vi "Double FFT Mesurament (Max Bin detection - Control - Windowing - Graph) test.vi"() -> ()   [LabVIEW 2014]
uses:
  <vilib>/Platform/TimedLoop/XDataNode/timing_clust.ctl
  <vilib>/Platform/TimedLoop/XDataNode/nitl_modes.ctl
  <vilib>/Platform/TimedLoop/XDataNode/wakeup.ctl
  <vilib>/rvi/Analysis/measure/FFT/simModelSupport/niFPGA FFT Streaming Sim Properties.ctl
  <vilib>/rvi/Analysis/measure/FFT/simModelSupport/niFPGA FFT Sim Stream Group Properties.ctl
  <vilib>/rvi/Analysis/measure/FFT/simModelSupport/niFPGA FFT Sim Types.ctl
  <vilib>/rvi/Analysis/measure/FFT/simModelSupport/niFpgaFFTSimArithmeticProperties.ctl
  <vilib>/rvi/Analysis/measure/FFT/simModelSupport/niFpgaFFTSimDfxp.ctl
  <vilib>/fxp/LVFixedPointQuantizationPolicyTypeDef.ctl
  <vilib>/rvi/Analysis/measure/FFT/XNode/niFpgaFFTButterflyDelays.ctl
  <vilib>/rvi/Emulation/niFpgaSctlEmulationGetInTimedLoop.vi
  <vilib>/rvi/Emulation/niFpgaEmulationReportErrorSimple.vi
  <vilib>/rvi/Emulation/niFpgaGetClockAttributes.vi
  <vilib>/rvi/Emulation/niFpgaCriticalErrorInLSC.vi
  <vilib>/rvi/Emulation/niFpgaEmulationIsFPGAContextNoSignature.vi
  <vilib>/rvi/errors/niFpgaSetErrorForExecOnDevCompSimple.vi
  <vilib>/rvi/eio/common/nirviEmuReportErrorAndStop.vi
  <vilib>/rvi/DataTransferAndStorage/Container/Common/niFpgaContainerGetUniqueNameForEmu.vi
  <vilib>/rvi/FIFO/Fifo_Resource/nirvififoEmulationSetSize.vi
  <vilib>/rvi/FIFO/Fifo_Resource/nirviFifoEmulationQueueMgr.vi
  <instcachedir>/0/nirviFifoEmulationQueueMgr_E5CAEC123FF24DC58D834DCA3CDAA9B5.lvgen/nirviFifoEmulationQueueMgr_E5CAEC123FF24DC58D834DCA3CDAA9B5_005.vi
  <vilib>/Utility/error.llb/Clear Errors.vi
  <vilib>/rvi/FIFO/Fifo_Resource/nirvififoEmulationCreateLock.vi
  <vilib>/rvi/Emulation/niFpgaProcessEmulError.vi
  <vilib>/rvi/FIFO/Fifo_Resource/nirvififoEmulationObtainLock.vi
  <vilib>/rvi/FIFO/Fifo_Resource/nirvififoEmulationReleaseLock.vi
  <vilib>/rvi/occurrence/nirviWaitOnOccurrenceBase.vi
  <vilib>/rvi/errors/nirviReportUnexpectedCaseInternalError.vi
  <vilib>/rvi/errors/nirviReportUnexpectedCaseInternalError (U32).vi
  <instcachedir>/0/nirviFifoEmulationQueueMgr_E5CAEC123FF24DC58D834DCA3CDAA9B5.lvgen/nirviFifoEmulationQueueMgr_E5CAEC123FF24DC58D834DCA3CDAA9B5_004.vi
  <vilib>/rvi/interface/RandomDataEmulation/niFpgaRandomDataHandleErrors.vi
  <vilib>/rvi/Memory/Memory_Emulation/niFpgaMemoryEmulationCacheClearOnFirstRun.vi
  <vilib>/rvi/Memory/Memory_Emulation/nirvimemoryEmulationManagerCache_MakeExclusive.vi
  <vilib>/rvi/Memory/Memory_Emulation/niFpgaMemoryEmulationValidateCache.vi
  <vilib>/rvi/Memory/Memory_Emulation/nirvimemoryEmulationManagerCache_InsertValue.vi
  <vilib>/rvi/Memory/Memory_Emulation/nirvimemoryEmulationManagerCache_ReleaseExclusive.vi
  <vilib>/rvi/Memory/Memory_Emulation/nirvimemoryEmulationManagerCache_GetValue.vi
  <vilib>/rvi/Memory/Memory_Emulation/nirvimemoryEmulationManagerCache_SetValue.vi
  <vilib>/rvi/FIFO/Fifo_Resource/nirvififoEmulationDetermineInputValidOut.vi
  <vilib>/rvi/Memory/Memory_Emulation/nirvimemoryFastEmulation.vi
  <vilib>/rvi/Memory/Memory_Emulation/nirvimemoryEmulation.vi
  <vilib>/rvi/Analysis/measure/FFT/simModelSupport/niFpgaFFTSimModelStreamingCore.vi
  <vilib>/rvi/eio/common/nirviEmuTemplateMethod_errors.vi
  <vilib>/Platform/TimedLoop/XDataNode/XDataNode.xnode
  <vilib>/rvi/DataTransferAndStorage/Container/XNode/niFpgaContainer.xnode
  <vilib>/rvi/FIFO/Fifo_Resource/nirvififoEmulationRead.vi
  <vilib>/rvi/interface/RandomDataEmulation/nirviRandomDataFpgaReadWriteTemplate.vi
  <vilib>/rvi/DataTransferAndStorage/Register/Emulation/niFpgaRegisterEmulation.vi
  <vilib>/rvi/FIFO/Fifo_Resource/nirvififoEmulationWrite.vi
  <vilib>/rvi/FIFO/Fifo_Resource/nirvififoEmulationGetNumberOfElementsToWrite.vi
  <vilib>/rvi/Analysis/measure/FFT/XNode/niFpgaFFT.xnode
  <vilib>/eio/EIOMethodNode/EIOMethodNode.xnode
  <vilib>/Platform/TimedLoop/XDataNode/XDNodeRunTimeDep.lvlib
panel:
  in  "snapshot":bool
  in  "first bin":i32=4
  in  "last bin":i32=251
  in  "lower limit 2":u32=682
  in  "lower limit 1":u32=57
  in  "upper limit 2":u32=1194
  in  "upper limit 1":u32=569
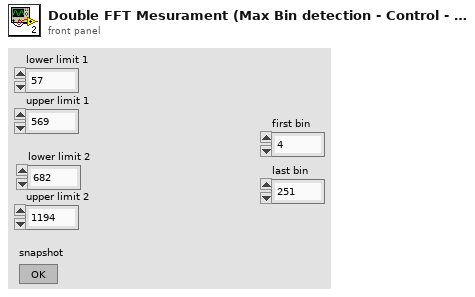
[diagram p1: front panel]
types:
  T1 = typedef "XDNodeRunTimeDep.lvlib/timing_clust.ctl" = cluster{"Expected End [f-1]":u64, "Actual End [f-1]":u64, "Finished Late? [f-1]":bool, "Expected End [i-1]":u64, "Actual End [i-1]":u64, "Finished Late? [i-1]":bool, "Expected Start [i]":u64, "Actual Start [i]":u64, "Expected Start [f]":u64, "Actual Start [f]":u64, "Source Name":string, "Structure Name":string, "Period":i64, "Deadline":i64, "Offset":i64, "Start":i64, "Priority":i32, "Timeout":i32, "Mode":T2, "Wakeup Reason":T3, "Error":errorcluster, "Source Type":string, "Secondary Source Type":string, "Global End Time":u64, "Global Start Time":u64, "Frame Duration":u64, "Iteration Duration":u64, "Assigned CPU":i32, "I/O Scan Engine Mode":u32}
  T2 = typedef "XDNodeRunTimeDep.lvlib/nitl_modes.ctl" = enum32{"No Change", "Process missed periods, maintain original phase", "Discard missed periods, maintain original phase", "Process missed periods, ignore original phase", "Discard missed periods, ignore original phase"}
  T3 = typedef "XDNodeRunTimeDep.lvlib/wakeup.ctl" = enum32{"Normal", "Aborted", "Asynchronous wakeup", "Timing source error", "Timed loop error", "Timeout"}
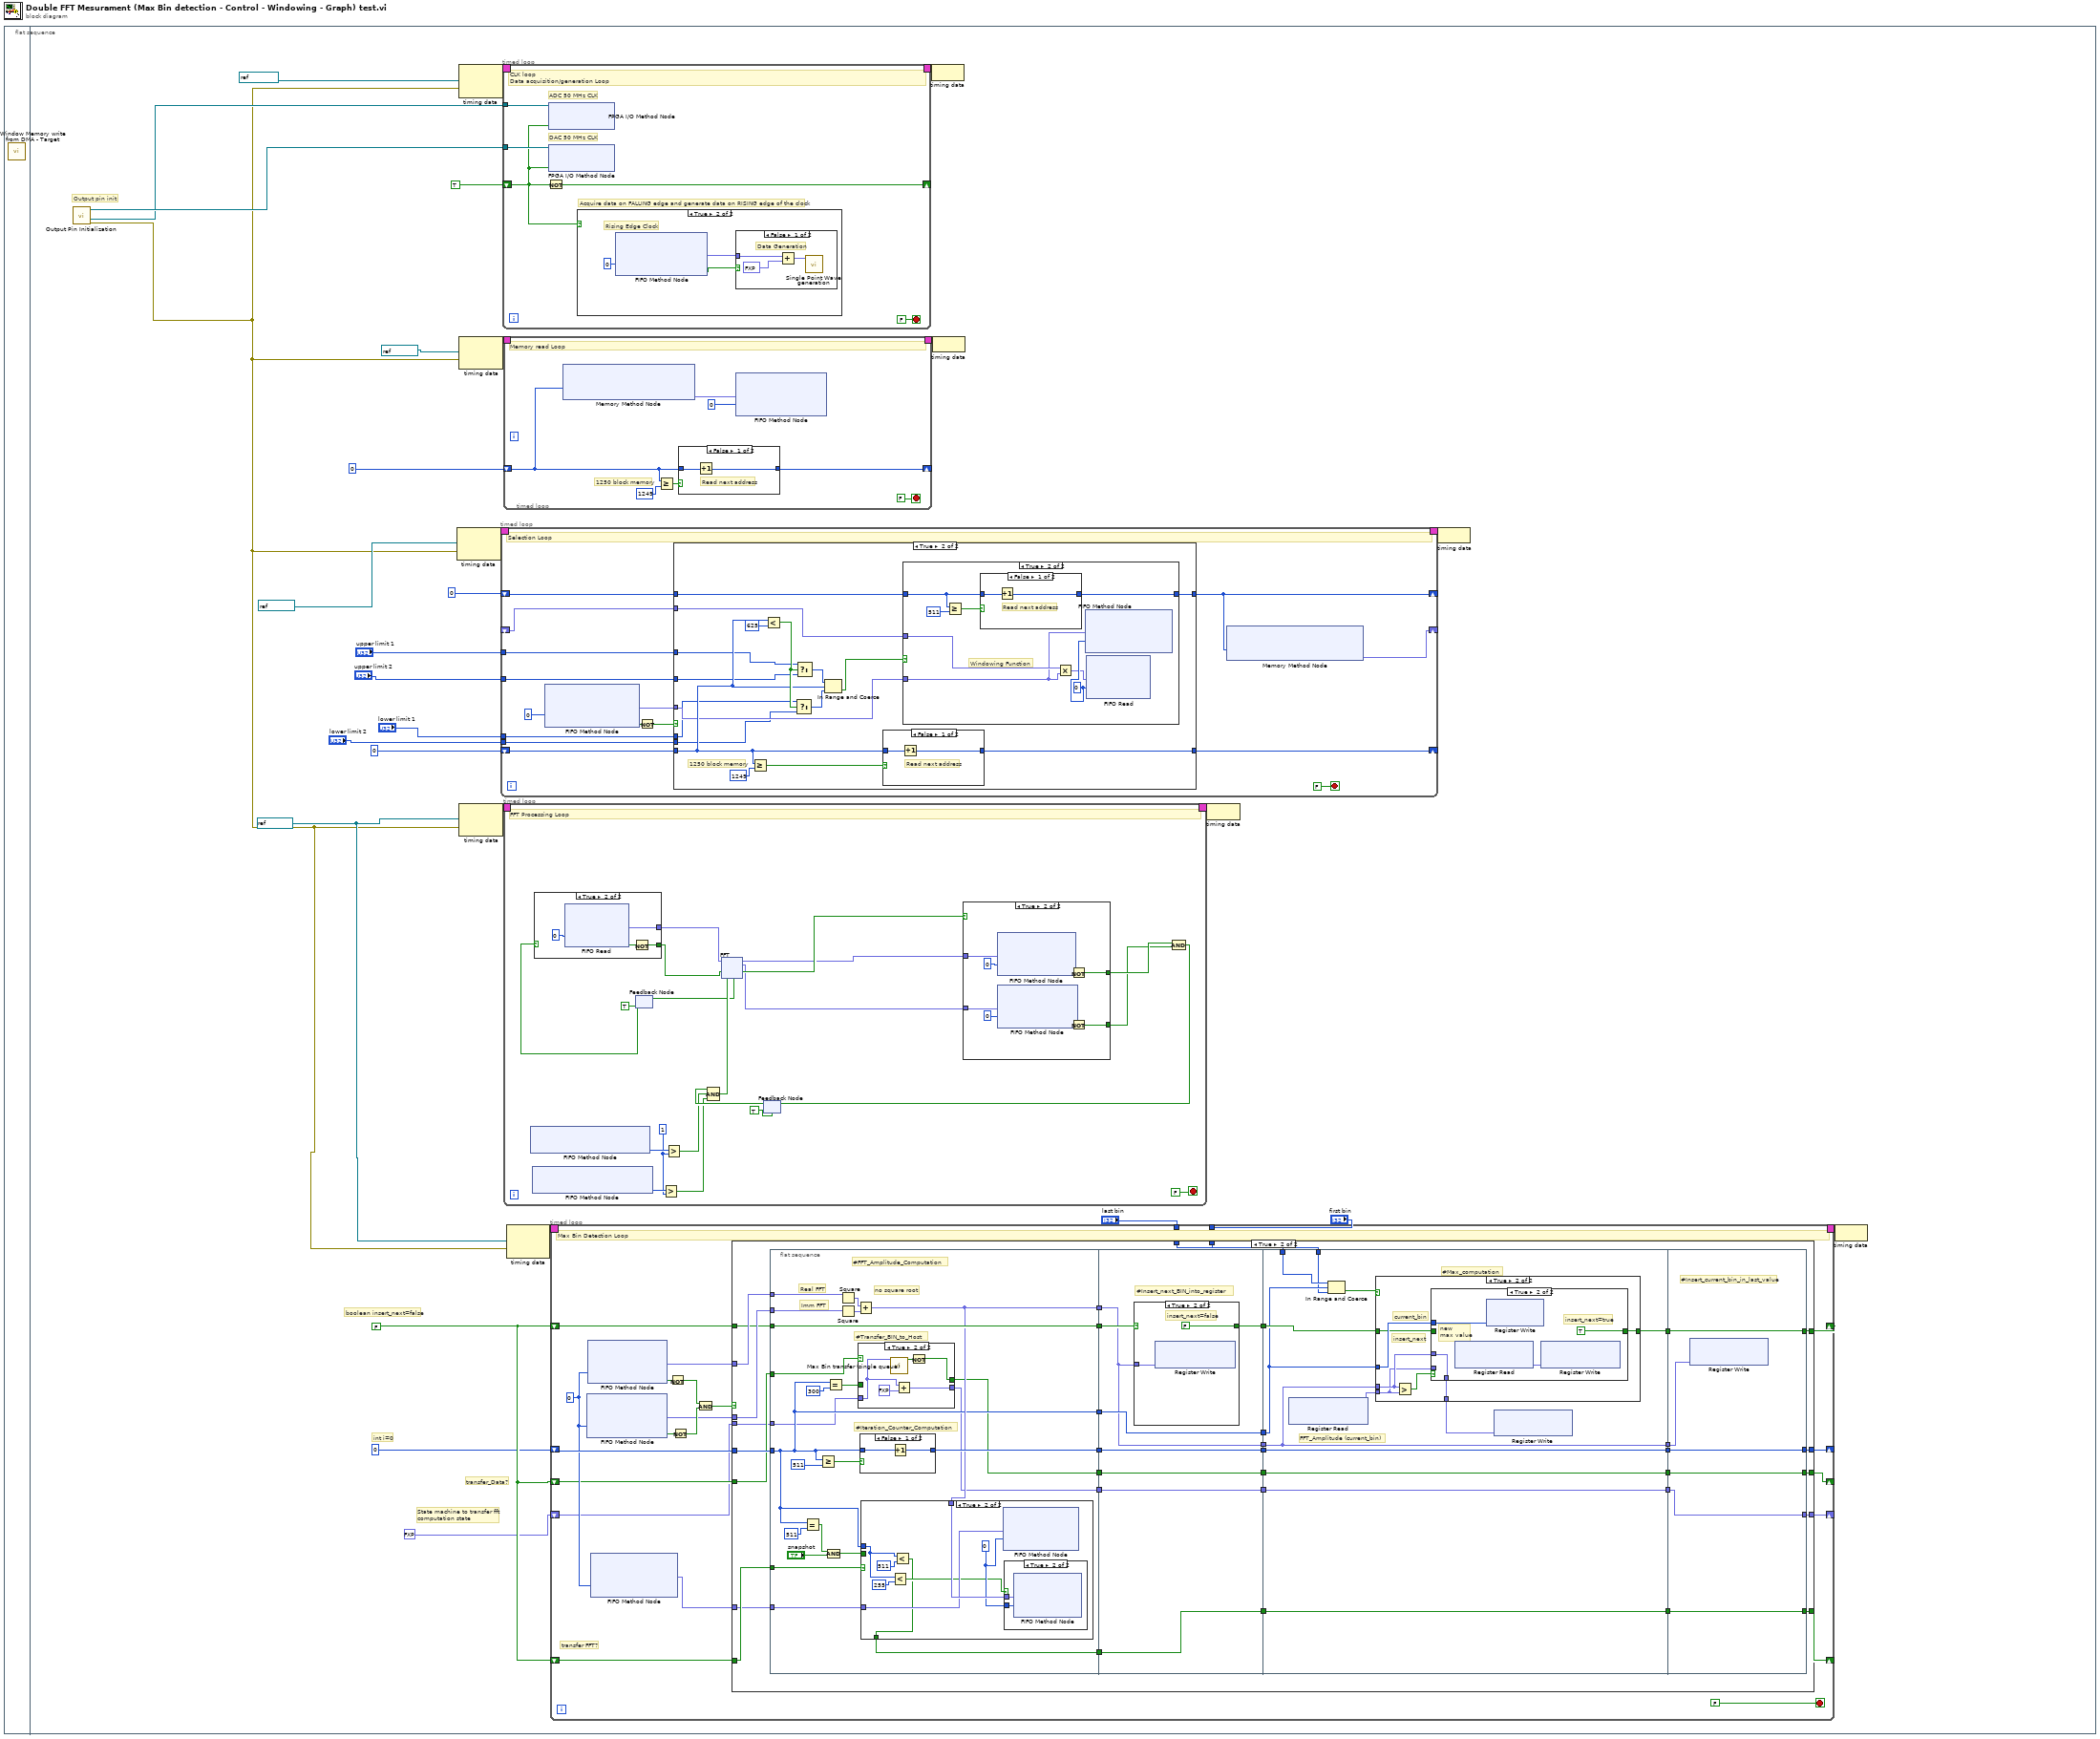
[diagram p0: block diagram]
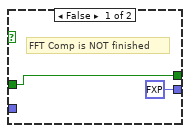
[diagram p5: hidden frame]
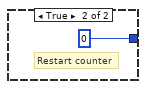
[diagram p6: hidden frame]
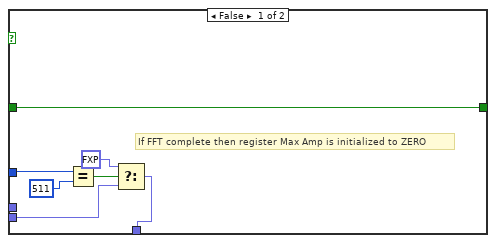
[diagram p8: hidden frame]
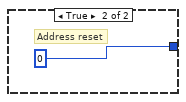
[diagram p12: hidden frame]
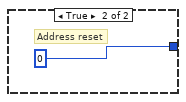
[diagram p13: hidden frame]
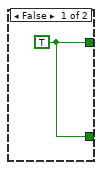
[diagram p14: hidden frame]
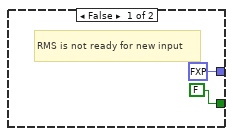
[diagram p15: hidden frame]
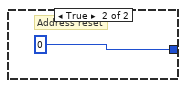
[diagram p16: hidden frame]
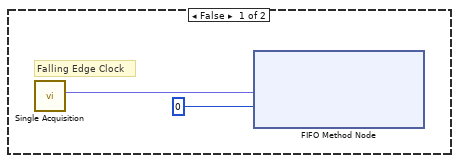
[diagram p17: hidden frame]
diagram:
  n1 = flat-sequence {
    frame #0 {
      n2 = call "Window Memory write from DMA - Target.vi"() -> ()  [unwired: 12 in]
    }
    frame #1 {
      w3 = FALSE
      w12 = refnum<k21> "50MHz" ("Source Name")
      # "State machine to transfer fft\ncomputation state"
      # "transfer_Data?"
      # "int i=0"
      # "boolean insert_next=false"
      # "Output pin init"
      n3 = call "Output Pin Initialization.vi"() -> ("error out"=w11:errorcluster, "I/O Out Clock DAC (pin16)"=w15:refnum<k21>, "I/O Out Clock ADC (pin17)"=w16:refnum<k21>)  [unwired: 8 in]
      n4 = node-c288(refnum<k21> "50MHz" ("Source Name"), w11) -> (w24:T1)
      n5 = node-c288(refnum<k21> "100MHz" ("Source Name"), w11) -> (w30:T1)
      n6 = node-c288(refnum<k21> "50MHz" ("Source Name"), w11) -> (w28:T1)
      n7 = node-c288(w12, w11) -> (w26:T1)
      n8 = timed-loop {
        timing: w24 -> [_]
        timing-out: [_] -> w23
        shift-right: [w207] -> _
        shift-left: u32 0 -> [w206]
        tunnel: "upper limit 1" -> [w201]
        tunnel: "upper limit 2" -> [w200]
        tunnel: "lower limit 1" -> [w199]
        tunnel: "lower limit 2" -> [w198]
        shift-right: [w194] -> _
        shift-left: u32 0 -> [w197]
        shift-right: [w195] -> _
        shift-left: _ -> [w196]
        stop <- FALSE stop-if-true
        # "Selection Loop"
        n9 = xnode ("FIFO Method Node")("Timeout"=0) -> ("Element"=w203:fxp<+/-,12,12>, "Timed Out?"=w204:bool)  [unwired: 1 in, 1 out]
        n10 = Not(x=w204) -> (.not. x?=w205:bool)
        n11 = case shown="True" w205 {
          tunnel: [w210 w225] -> w207
          tunnel: w206 -> [w210 w220]
          tunnel: w203 -> [_ w218]
          tunnel: w201 -> [_ w217]
          tunnel: w200 -> [_ w216]
          tunnel: w199 -> [_ w215]
          tunnel: w198 -> [_ w214]
          tunnel: w197 -> [w209 w211]
          tunnel: [w209 w213] -> w194
          tunnel: w196 -> [_ w212]
          frame False {
          }
          frame True {
            # "1250 block memory"
            n12 = Greater Or Equal?(x=w220, y=u32 1249) -> (x >= y?=w226:bool)
            n13 = Less?(x=w220, y=u32 625) -> (x < y?=w221:bool)
            n14 = Select(t=w215, s=w221, f=w214) -> (s? t:f=w223:u32)
            n15 = Select(t=w217, s=w221, f=w216) -> (s? t:f=w224:u32)
            n16 = In Range and Coerce(upper limit=w224, x=w220, lower limit=w223) -> (In Range?=w219:bool)  [unwired: 1 out]
            n17 = case shown="False" w226 {
              tunnel: w220 -> [w241 _]
              tunnel: [w240 u32 0] -> w225
              frame False {
                # "Read next address"
                n18 = Increment(x=w241) -> (x+1=w240:u32)
              }
              frame True {
                # "Address reset"
              }
            }
            n19 = case shown="True" w219 {
              tunnel: w218 -> [_ w229]
              tunnel: w211 -> [w228 w234]
              tunnel: [w228 w236] -> w213
              tunnel: w212 -> [_ w232]
              frame False {
              }
              frame True {
                w231 = 0 ("Timeout")
                # "Windowing Function"
                n20 = Greater Or Equal?(x=w234, y=u32 511) -> (x >= y?=w235:bool)
                n21 = case shown="False" w235 {
                  tunnel: w234 -> [w238 _]
                  tunnel: [w237 u32 0] -> w236
                  frame False {
                    # "Read next address"
                    n22 = Increment(x=w238) -> (x+1=w237:u32)
                  }
                  frame True {
                    # "Address reset"
                  }
                }
                n23 = Multiply(x=w232, y=w229) -> (x*y=w230:fxp<+/-,12,12>)
                n24 = xnode ("FIFO Method Node")("Element"=w229, "Timeout"=w231) -> ()  [unwired: 1 in, 2 out]
                n25 = xnode ("FIFO Read")("Element"=w230, "Timeout"=w231) -> ()  [unwired: 1 in, 2 out]
              }
            }
          }
        }
        n26 = xnode ("Memory Method Node")("Address"=w194) -> ("Data"=w195:fxp<+,8,1>)  [unwired: 1 in, 1 out]
      }
      n27 = timed-loop {
        timing: w30 -> [_]
        timing-out: [_] -> w29
        shift-right: [w337] -> _
        shift-left: TRUE -> [w335]
        tunnel: w15 -> [w339]
        tunnel: w16 -> [w336]
        stop <- FALSE stop-if-true
        # "DAC 50 MHz CLK"
        # "Acquire data on FALLING edge and generate data on RISING edge of the clock"
        # "ADC 50 MHz CLK"
        # "CLK loop\nData acquisition/generation Loop"
        n28 = Not(x=w335) -> (.not. x?=w337:bool)
        n29 = xnode "FPGA I/O Method Node"("FPGA I/O In"=w339, "Data"=w335) -> ()  [unwired: 1 out]
        n30 = xnode "FPGA I/O Method Node"("FPGA I/O In"=w336, "Data"=w335) -> ()  [unwired: 1 out]
        n31 = case shown="True" w335 {
          frame False {
            # "Falling Edge Clock"
            n32 = call "Single Acquisition.vi"() -> ("Out"=w341:fxp<+/-,12,12>)  [unwired: 10 in, 1 out]
            n33 = xnode ("FIFO Method Node")("Element"=w341, "Timeout"=0) -> ()  [unwired: 1 in, 2 out]
          }
          frame True {
            # "Rising Edge Clock"
            n34 = xnode ("FIFO Method Node")("Timeout"=0) -> ("Element"=w342:fxp<+/-,12,12>, "Timed Out?"=w343:bool)  [unwired: 1 in, 1 out]
            n35 = case shown="False" w343 {
              tunnel: w342 -> [w347 _]
              frame False {
                # "Data Generation"
                n36 = Add(x=w347, y=fxp<+,12,12> 2048.0) -> (x+y=w345:fxp<+/-,14,14>)
                n37 = call "Single Point Wave generation.vi"("Data To Write"=w345) -> ()  [unwired: 10 in, 1 out]
              }
              frame True {
                # "FPGA memory slow"
              }
            }
          }
        }
      }
      n38 = timed-loop {
        timing: w28 -> [_]
        timing-out: [_] -> w27
        shift-right: [w322] -> _
        shift-left: u32 0 -> [w320]
        stop <- FALSE stop-if-true
        # "1250 block memory"
        # "Memory read Loop"
        n39 = xnode ("Memory Method Node")("Address"=w320) -> ("Data"=w319:fxp<+/-,12,12>)  [unwired: 1 in, 1 out]
        n40 = Greater Or Equal?(x=w320, y=u32 1249) -> (x >= y?=w323:bool)
        n41 = case shown="False" w323 {
          tunnel: w320 -> [w326 _]
          tunnel: [w325 u32 0] -> w322
          frame False {
            # "Read next address"
            n42 = Increment(x=w326) -> (x+1=w325:u32)
          }
          frame True {
            # "Address reset"
          }
        }
        n43 = xnode ("FIFO Method Node")("Element"=w319, "Timeout"=0) -> ()  [unwired: 1 in, 2 out]
      }
      n44 = timed-loop {
        timing: w26 -> [_]
        timing-out: [_] -> w25
        stop <- FALSE stop-if-true
        w252 = u32 1 ("y")
        # "FFT Processing Loop"
        n45 = xnode ("FIFO Method Node")() -> ("Number of Elements to Write"=w254:u32)  [unwired: 1 in, 1 out]
        n46 = xnode ("FIFO Method Node")() -> ("Number of Elements to Write"=w253:u32)  [unwired: 1 in, 1 out]
        n47 = feedback #1(TRUE ("ready for input")) -> (w269:bool)
        n48 = case shown="True" w269 {
          tunnel: [FALSE w310] -> w263
          tunnel: [fxp<+/-,12,12> 0.0 ("Element") w307] -> w264
          frame False {
            # "RMS is not ready for new input"
          }
          frame True {
            n49 = xnode ("FIFO Read")("Timeout"=0) -> ("Element"=w307:fxp<+/-,12,12>, "Timed Out?"=w309:bool)  [unwired: 1 in, 1 out]
            n50 = Not(x=w309) -> (.not. x?=w310:bool)
          }
        }
        n51 = Greater?(x=w253, y=w252) -> (0:w250:bool)
        n52 = Greater?(x=w254, y=w252) -> (0:w251:bool)
        n53 = feedback #2(TRUE) -> (w265:bool)
        n54 = Compound Arithmetic op=AND(w265, w251, w250) -> (w262:bool)
        n55 = xnode "FFT"("real data in"=w264, "input valid"=w263, "ready for output"=w262) -> ("ready for input"=w261:bool, "real data out"=w259:fxp<+/-,22,22>, "imaginary data out"=w258:fxp<+/-,22,22>, "output valid"=w260:bool)  [unwired: 2 in, 1 out]
        n56 = feedback-in #1(w261) -> ()
        n57 = case shown="True" w260 {
          tunnel: w259 -> [_ w304]
          tunnel: w258 -> [_ w303]
          tunnel: [w296 w302] -> w257
          tunnel: [w296 w301] -> w256
          frame False {
            w296 = TRUE
          }
          frame True {
            n58 = xnode ("FIFO Method Node")("Element"=w304, "Timeout"=0) -> ("Timed Out?"=w297:bool)  [unwired: 1 in, 1 out]
            n59 = xnode ("FIFO Method Node")("Element"=w303, "Timeout"=0) -> ("Timed Out?"=w298:bool)  [unwired: 1 in, 1 out]
            n60 = Not(x=w297) -> (.not. x?=w302:bool)
            n61 = Not(x=w298) -> (.not. x?=w301:bool)
          }
        }
        n62 = Compound Arithmetic op=AND(w257, w256) -> (w255:bool)
        n63 = feedback-in #2(w255) -> ()
      }
      n64 = node-c288(w12, w11) -> (w22:T1)
      n65 = timed-loop {
        shift-right: [w44] -> _
        shift-left: 0 ("Timeout") -> [w45]
        shift-right: [w42] -> _
        shift-left: w3 -> [w43]
        timing: w22 -> [_]
        timing-out: [_] -> w21
        tunnel: "last bin" -> [w40]
        tunnel: "first bin" -> [w39]
        shift-right: [w38] -> _
        shift-left: w3 -> [w37]
        shift-right: [w33] -> _
        shift-left: w3 -> [w34]
        shift-right: [w31] -> _
        shift-left: fxp<+,2,2> 0.0 ("Timeout") -> [w32]
        stop <- FALSE stop-if-true
        w36 = 0 ("Timeout")
        # "transfer FFT?"
        # "Max Bin Detection Loop"
        n66 = xnode ("FIFO Method Node")("Timeout"=w36) -> ("Element"=w46:fxp<+/-,22,22>, "Timed Out?"=w51:bool)  [unwired: 1 in, 1 out]
        n67 = xnode ("FIFO Method Node")("Timeout"=w36) -> ("Element"=w47:fxp<+/-,22,22>, "Timed Out?"=w52:bool)  [unwired: 1 in, 1 out]
        n68 = xnode ("FIFO Method Node")("Timeout"=w36) -> ("Element"=w35:fxp<+/-,12,12>)  [unwired: 1 in, 2 out]
        n69 = Not(x=w52) -> (.not. x?=w50:bool)
        n70 = Not(x=w51) -> (.not. x?=w49:bool)
        n71 = And(x=w50, y=w49) -> (x .and. y?=w48:bool)
        n72 = case shown="True" w48 {
          tunnel: w47 -> [_ w92]
          tunnel: w46 -> [_ w91]
          tunnel: w45 -> [w57 w89]
          tunnel: [w57 w76] -> w44
          tunnel: w43 -> [w56 w83]
          tunnel: [w56 w78] -> w42
          tunnel: w40 -> [_ w75]
          tunnel: w39 -> [_ w74]
          tunnel: [w55 w70] -> w38
          tunnel: w37 -> [w55 w69]
          tunnel: w35 -> [_ w68]
          tunnel: w34 -> [w54 w67]
          tunnel: [w54 w66] -> w33
          tunnel: w32 -> [w53 w62]
          tunnel: [w53 w58] -> w31
          frame False {
            # "Data are NOT ready in Target Real FFT and Target Imm FFT FIFOs"
          }
          frame True {
            n73 = flat-sequence {
              tunnel: w92 -> [w112]
              tunnel: w91 -> [w113]
              tunnel: [w103] -> w90
              tunnel: w89 -> [w99]
              tunnel: [w111] -> w88
              tunnel: [w99] -> w85
              tunnel: [w108] -> w84
              tunnel: w83 -> [w108]
              tunnel: [w101] -> w73
              tunnel: w69 -> [w100]
              tunnel: w68 -> [w98]
              tunnel: w67 -> [w97]
              tunnel: [w95] -> w65
              tunnel: w62 -> [w94]
              tunnel: [w93] -> w61
              tunnel: w90 -> [w141]
              tunnel: w88 -> [w144]
              tunnel: [w144] -> w87
              tunnel: w85 -> [w142]
              tunnel: w84 -> [w143]
              tunnel: [w142] -> w82
              tunnel: [w141] -> w81
              tunnel: [w140] -> w80
              tunnel: w73 -> [w139]
              tunnel: [w139] -> w71
              tunnel: w65 -> [w138]
              tunnel: [w138] -> w64
              tunnel: w61 -> [w137]
              tunnel: [w137] -> w59
              tunnel: w87 -> [w160]
              tunnel: [w160] -> w86
              tunnel: w82 -> [w155]
              tunnel: w81 -> [w157]
              tunnel: w80 -> [w158]
              tunnel: [w157] -> w79
              tunnel: [w156] -> w77
              tunnel: w75 -> [w152]
              tunnel: w74 -> [w151]
              tunnel: [w150] -> w72
              tunnel: w71 -> [w150]
              tunnel: w64 -> [w149]
              tunnel: [w149] -> w63
              tunnel: [w148] -> w60
              tunnel: w59 -> [w148]
              tunnel: w86 -> [w184]
              tunnel: w79 -> [w186]
              tunnel: w77 -> [w185]
              tunnel: [w185] -> w78
              tunnel: [w184] -> w76
              tunnel: [w183] -> w70
              tunnel: w72 -> [w183]
              tunnel: [w182] -> w66
              tunnel: w63 -> [w182]
              tunnel: w60 -> [w181]
              tunnel: [w181] -> w58
              frame #0 {
                # "no square root"
                # "#Transfer_BIN_to_Host"
                # "#Iteration_Counter_Computation"
                # "#FFT_Amplitude_Computation"
                # "Imm FFT"
                # "Real FFT"
                n74 = Equal?(x=w99, y=511) -> (x = y?=w104:bool)
                n75 = Greater Or Equal?(x=w99, y=511) -> (x >= y?=w109:bool)
                n76 = Equal?(x=w99, y=300) -> (x = y?=w96:bool)
                n77 = Compound Arithmetic op=AND(w104, "snapshot") -> (w102:bool)
                n78 = Square(x=w112) -> (x^2=w115:fxp<+,43,43>)
                n79 = Square(x=w113) -> (x^2=w114:fxp<+,43,43>)
                n80 = Add(x=w115, y=w114) -> (x+y=w103:fxp<+,44,44>)
                n81 = case shown="True" w97 {
                  tunnel: w96 -> [w128 _]
                  tunnel: [w128 w132] -> w95
                  tunnel: w94 -> [_ w131]
                  tunnel: [fxp<+,2,2> 0.0 w129] -> w93
                  frame False {
                    # "FFT Comp is NOT finished"
                  }
                  frame True {
                    n82 = call "Max Bin transfer (single queue).vi"("Enum"=w131) -> ("END?"=w133:bool)  [unwired: 10 in]
                    n83 = Add(x=w131, y=fxp<+,2,2> 1.0) -> (x+y=w129:fxp<+,2,2>)
                    n84 = Not(x=w133) -> (.not. x?=w132:bool)
                  }
                }
                n85 = case shown="False" w109 {
                  tunnel: w99 -> [w134 _]
                  tunnel: [w135 0 ("Timeout")] -> w111
                  frame False {
                    n86 = Increment(x=w134) -> (x+1=w135:i32)
                  }
                  frame True {
                    # "Restart counter"
                  }
                }
                n87 = case shown="True" w100 {
                  tunnel: w103 -> [_ w124]
                  tunnel: w102 -> [w116 _]
                  tunnel: [w116 w117] -> w101
                  tunnel: w99 -> [_ w118]
                  tunnel: w98 -> [_ w121]
                  frame False {
                  }
                  frame True {
                    w122 = 0 ("Timeout")
                    n88 = Less?(x=w118, y=255) -> (x < y?=w120:bool)
                    n89 = Less?(x=w118, y=511) -> (x < y?=w117:bool)
                    n90 = xnode ("FIFO Method Node")("Element"=w121, "Timeout"=w122) -> ()  [unwired: 1 in, 2 out]
                    n91 = case shown="True" w120 {
                      tunnel: w124 -> [_ w126]
                      tunnel: w122 -> [_ w125]
                      frame False {
                      }
                      frame True {
                        n92 = xnode ("FIFO Method Node")("Element"=w126, "Timeout"=w125) -> ()  [unwired: 1 in, 2 out]
                      }
                    }
                  }
                }
              }
              frame #1 {
                # "#Insert_next_BIN_into_register"
                n93 = case shown="True" w143 {
                  selector: w143 -> [w145 _]
                  tunnel: [w145 FALSE] -> w140
                  tunnel: w141 -> [_ w146]
                  frame False {
                  }
                  frame True {
                    # "insert_next=false"
                    n94 = xnode ("Register Write")("Data"=w146) -> ()  [unwired: 1 in, 1 out]
                  }
                }
              }
              frame #2 {
                # "FFT_Amplitude (current_bin)"
                # "#Max_computation"
                n95 = xnode ("Register Read")() -> ("Data"=w154:fxp<+,44,44>)  [unwired: 1 in, 1 out]
                n96 = In Range and Coerce(upper limit=w152, x=w155, lower limit=w151) -> (In Range?=w159:bool)  [unwired: 1 out]
                n97 = case shown="True" w159 {
                  tunnel: w157 -> [_ w173]
                  tunnel: w155 -> [w165 w172]
                  tunnel: w158 -> [w167 w171]
                  tunnel: [w167 w170] -> w156
                  tunnel: w154 -> [w163 w168]
                  tunnel: [w161 w169] -> w153
                  frame False {
                    # "If FFT complete then register Max Amp is initialized to ZERO"
                    n98 = Equal?(x=w165, y=511) -> (x = y?=w166:bool)
                    n99 = Select(t=fxp<+,44,44> 0.0, s=w166, f=w163) -> (s? t:f=w161:fxp<+,44,44>)
                  }
                  frame True {
                    # "insert_next"
                    # "current_bin"
                    n100 = Greater?(x=w173, y=w168) -> (0:w174:bool)
                    n101 = case shown="True" w174 {
                      tunnel: w173 -> [_ w177]
                      tunnel: w172 -> [_ w180]
                      tunnel: w171 -> [w176 _]
                      tunnel: [w176 TRUE] -> w170
                      tunnel: [w175 w177] -> w169
                      tunnel: w168 -> [w175 _]
                      frame False {
                        # "Old value is re-written"
                      }
                      frame True {
                        # "new\nmax value"
                        # "insert_next=true"
                        n102 = xnode ("Register Read")() -> ("Data"=w178:fxp<+,44,44>)  [unwired: 1 in, 1 out]
                        n103 = xnode ("Register Write")("Data"=w180) -> ()  [unwired: 1 in, 1 out]
                        n104 = xnode ("Register Write")("Data"=w178) -> ()  [unwired: 1 in, 1 out]
                      }
                    }
                  }
                }
                n105 = xnode ("Register Write")("Data"=w153) -> ()  [unwired: 1 in, 1 out]
              }
              frame #3 {
                # "#Insert_current_bin_in_last_value"
                n106 = xnode ("Register Write")("Data"=w186) -> ()  [unwired: 1 in, 1 out]
              }
            }
          }
        }
      }
      n107 = node-c288(w29) -> ()
      n108 = node-c288(w27) -> ()
      n109 = node-c288(w25) -> ()
      n110 = node-c288(w23) -> ()
      n111 = node-c288(w21) -> ()
    }
  }
